vi "Get Control Information.vi"(8 "error in (no error)":errorcluster, 11 "Numeric in":refnum<class "Numeric.lvclass">) -> (0 "error out":errorcluster, 2 "Control Information":string[][](array[string]), 3 "Numeric out":refnum<class "Numeric.lvclass">)   [LabVIEW 2017, in "Localization.lvlib" / "Numeric.lvclass"]
doc: "VI for override that is supposed to do go throgh the process for each control type and pull out the information that is necessary for each control.\n\nChoose Movement Consulting, LLC"
uses:
  Numeric.lvclass
  C:/Apps/CMC/OpenSource/Localization/Control Info/Control Info.lvclass
  Localization.lvlib
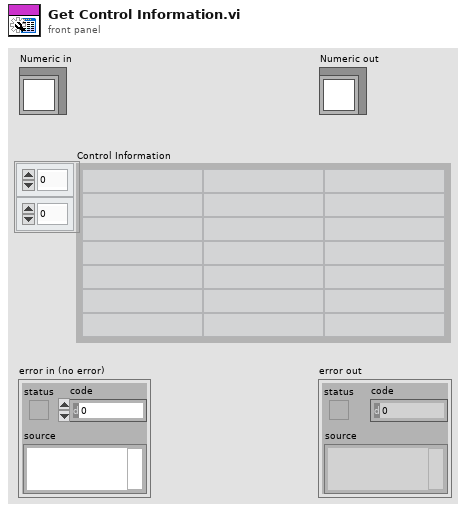
[diagram p1: front panel]
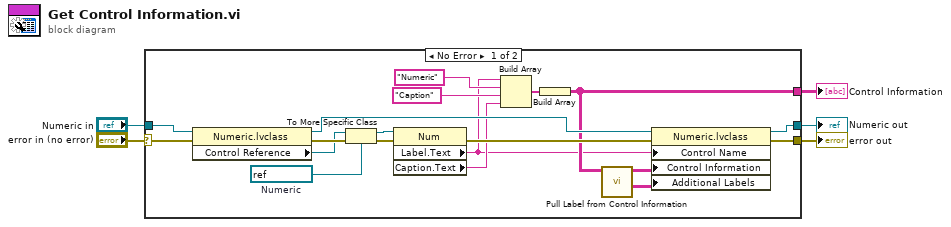
[diagram p0: block diagram]
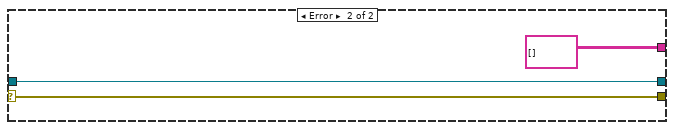
[diagram p2: hidden frame]
diagram:
  n1 = case shown="No Error" "error in (no error)" {
    selector: "error in (no error)" -> [w17 w27]
    tunnel: [w13 w27] -> w4
    tunnel: "Numeric in" -> [w16 w26]
    tunnel: [w9 string[][] []] -> w2
    tunnel: [w11 w26] -> w1
    frame No Error {
      w24 = refnum<vi> refnum  # Numeric
      n2 = property class="Numeric.lvclass"(reference=w16, error in=w17) -> (reference out=w12:refnum<class "Numeric.lvclass">, error out=w18:errorcluster, "Control Reference"=w15:refnum<vi>)
      n3 = To More Specific Class(target class=w24, reference=w15, error in=w18) -> (specific class reference=w23:refnum<vi>, error out=w19:errorcluster)
      n4 = property class="Num"(reference=w23, error in=w19) -> (error out=w14:errorcluster, "Label.Text"=w6:string, "Caption.Text"=w10:string)  [unwired: 1 out]
      n5 = Build Array(w6, "Numeric", "Caption", w10) -> (w20:string[])
      n6 = Build Array(w20) -> (w9:string[][])
      n7 = call "Pull Label from Control Information.vi"("Control Caption Table"=w9) -> ("Additional Labels"=w7:string[][], "Control Information"=w8:string[][])  [unwired: 9 in]
      n8 = property class="Numeric.lvclass"(reference=w12, error in=w14, "Control Name"=w6, "Control Information"=w8, "Additional Labels"=w7) -> (reference out=w11:refnum<class "Numeric.lvclass">, error out=w13:errorcluster)
    }
    frame Error {
    }
  }
  "error out" <- w4
  "Numeric out" <- w1
  "Control Information" <- w2
